vi "CRYGet Curve Library Data Name.vi"(6 "nData":i32[](array[numeric]), 7 "Step No.":i32, 8 "sData":string, 9 "sOption":string, 10 "sAction":string, 11 "Type":enum16{"Curves", "Values", "Results", "WFM"}(ring)) -> (0 "Index":i32[](array[numeric]), 1 "nStep No":i32[](array[numeric]), 2 "sNames":string[](array[string]), 3 "Type Out":string[](array[string]))   [LabVIEW 2013]
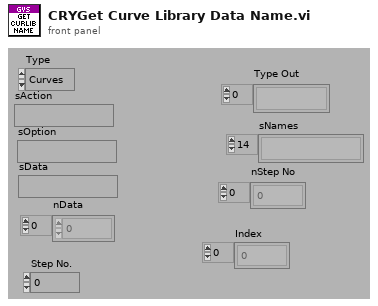
[diagram p1: front panel]
types:
  T1 = typedef "CRYData Cluster.ctl" = cluster{"Name":string, "Curve":cluster{"x":dbl, "y":dbl, "z":dbl}[], "X data":u16, "Y data":u16, "Z data":u16, "X axis":u16, "Y axis":u16, "Z axis":u16, "X unit":string, "Y unit":string, "Z unit":string, "X dB ref":dbl, "Y dB ref":dbl, "Z dB ref":dbl, "single val":bool, "protected":bool, "display X":bool, "display Y":bool, "display Z":bool, "Test Info":string, "Step No.":i32, "Plot Settings":cluster{"Color":u32, "Interpolation":u8, "Point Style":u8, "Line Style":u8, "Point Color":u32, "Line Width":u8, "Bar Plot Style":u8, "Fill To":i16}, "AutoProtect":bool}
  T2 = typedef "CRYWaveform Cluster.ctl" = cluster{"Waveform":cluster{"X0":dbl, "dX":dbl, "Y":sgl[]}, "X data":u16, "Y data":u16, "Y axis":u16, "X unit":string, "Y unit":string, "Y dB ref":dbl, "display Y":bool, "display X":bool, "Overload?":bool, "Test Info":string, "Step No.":i32, "Name":string, "protected":bool, "Sqc history":string[], "Signal Channel ID":i32, "Plot Settings":cluster{"Color":u32, "Interpolation":u8, "Point Style":u8, "Line Style":u8, "Point Color":u32, "Line Width":u8, "Bar Plot Style":u8, "Fill To":i16}, "AutoProtect":bool}
  T3 = typedef "CRYResult Cluster.ctl" = cluster{"Name":string, "Margin":dbl, "unit":string, "Verdict":bool, "Limit":string, "Max/Min":string, "protected":bool, "Step No.":i32, "Test Info":string, "AutoProtect":bool}
  T4 = typedef "CRYStimulus Test Infor Cluster.ctl" = cluster{"Stimulus Type":string, "Signal Type":string, "In/Out":bool, "FAPS":cluster{"freq":dbl, "ampl":dbl, "cycles":dbl, "samples":i32}[], "Sampling Rate":dbl, "Samples":i32, "Analysis Param":string, "Resolution":u16, "Steps":u32, "Analysis Value":dbl[], "Diff Freq":dbl, "FStart":dbl, "FStop":dbl, "Calibration Param":string, "Anti Alias":dbl, "Level Out1":dbl, "Level Out2":dbl, "EQ":bool}
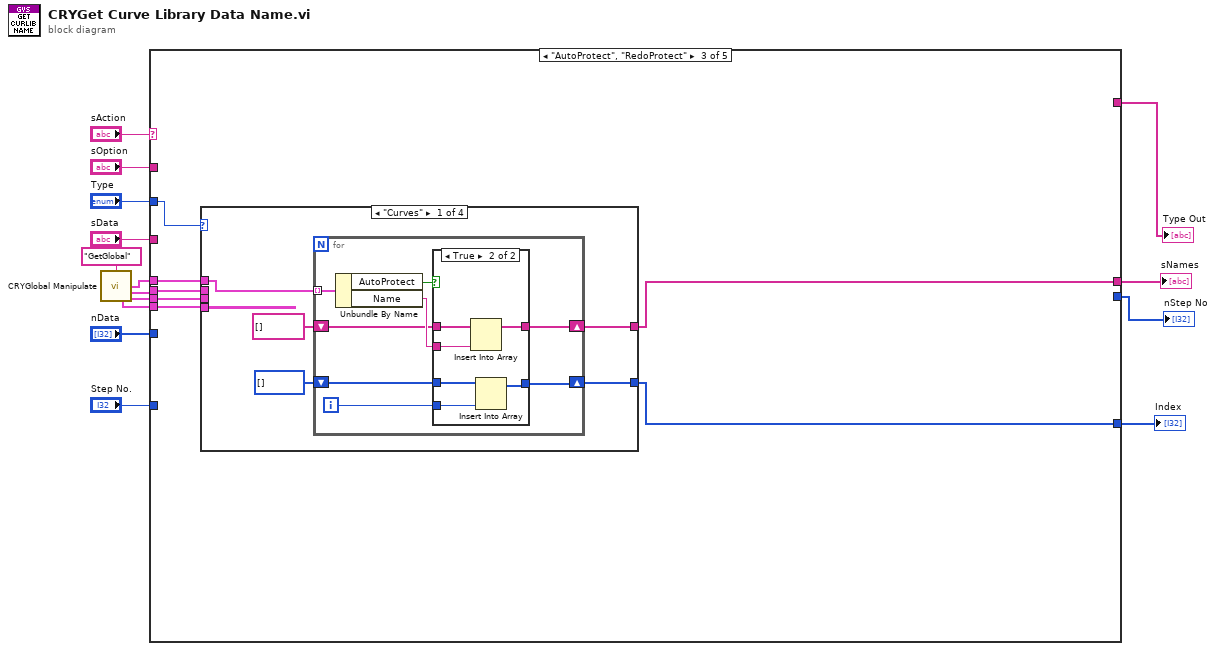
[diagram p0: block diagram]
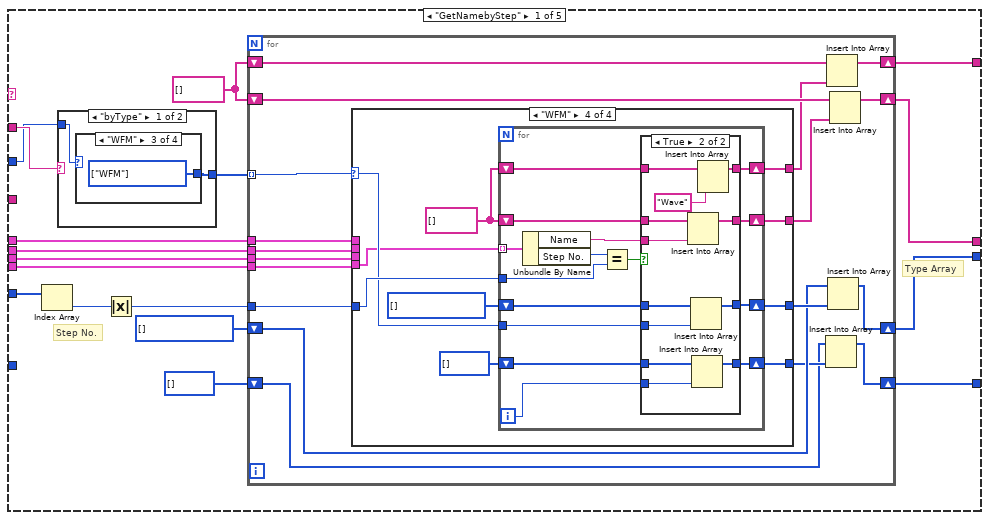
[diagram p2: hidden frame]
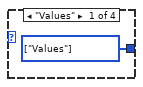
[diagram p3: hidden frame]
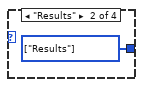
[diagram p4: hidden frame]
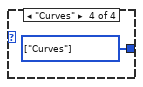
[diagram p5: hidden frame]
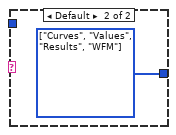
[diagram p6: hidden frame]
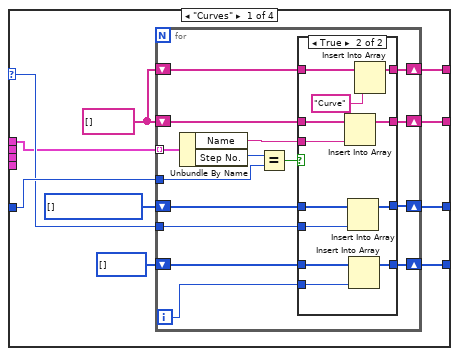
[diagram p7: hidden frame]
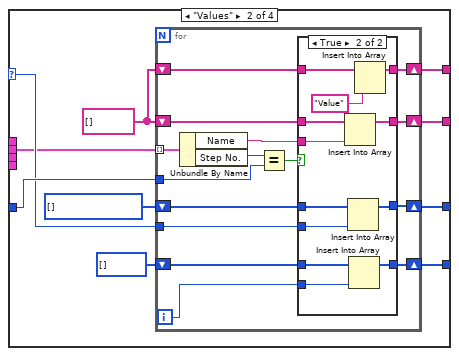
[diagram p9: hidden frame]
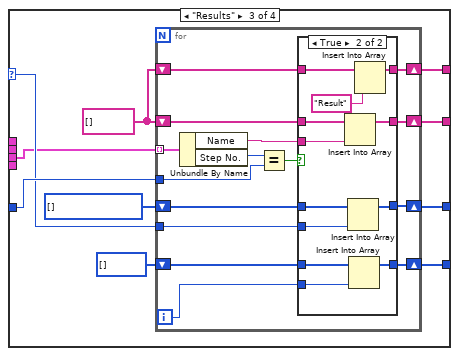
[diagram p11: hidden frame]
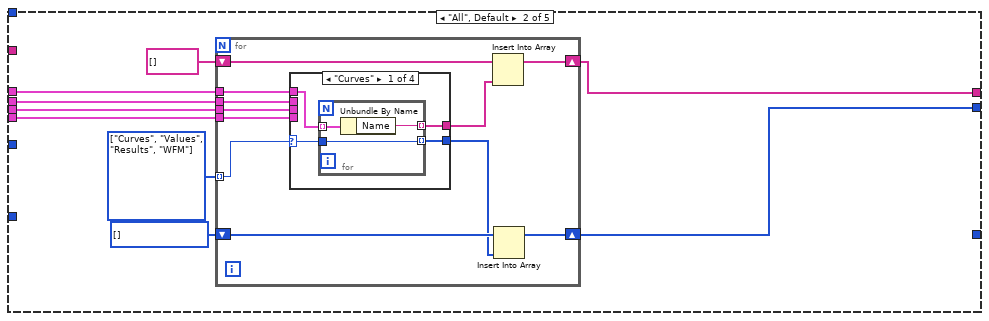
[diagram p14: hidden frame]
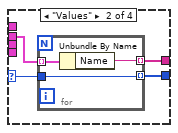
[diagram p15: hidden frame]
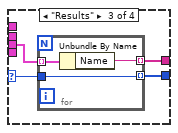
[diagram p16: hidden frame]
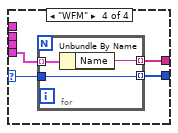
[diagram p17: hidden frame]
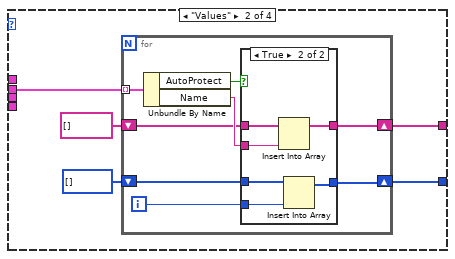
[diagram p19: hidden frame]
diagram:
  n1 = call "CRYGlobal Manipulate.vi"("sAction"="GetGlobal") -> ("Curves Out"=w1:T1[], "Values Out"=w2:T1[], "WFM Out"=w4:T2[], "Results Out"=w5:T3[])  [unwired: 8 in, 3 out]
  n2 = case shown="\"AutoProtect\", \"RedoProtect\"" "sAction" {
    tunnel: "Type" -> [w25 _ w274 _ w532]
    tunnel: "sOption" -> [w26 _ _ _ w536]
    tunnel: "nData" -> [w31 _ _ w367 w531]
    tunnel: "sData" -> [_ _ _ _ w535]
    tunnel: [w29 w228 w275 w368 w534] -> w11
    tunnel: [w27 w226 _ i32[] [] w533] -> w10
    tunnel: [w23 _ w276 _ _] -> w9
    tunnel: "Step No." -> [_ _ _ w366 _]
    tunnel: [w21 _ _ _ _] -> w7
    tunnel: w2 -> [w20 w225 w273 w365 w530]
    tunnel: w5 -> [w19 w224 w272 w364 w529]
    tunnel: w4 -> [w18 w223 w271 w363 w528]
    tunnel: w1 -> [w17 w222 w270 w362 w527]
    frame "GetNamebyStep" {
      w28 = enum16{"Curves", "Values", "Results", "WFM"}[] [] items=["Curves", "Values", "Results", "WFM"]
      w22 = string[] []
      # "Type Array"
      # "Step No."
      n3 = Index Array(array=w31) -> (element=w30:i32)  [unwired: 1 in]
      n4 = case shown="\"byType\"" w26 {
        tunnel: [w33 w39] -> w32
        tunnel: w25 -> [w34 _]
        frame "byType" {
          n5 = case shown="\"WFM\"" w34 {
            tunnel: [w35 w36 w37 w38] -> w33
            frame "Values" {
              w35 = enum16{"Curves", "Values", "Results", "WFM"}[] [enum."Values"] items=["Curves", "Values", "Results", "WFM"]
            }
            frame "Results" {
              w36 = enum16{"Curves", "Values", "Results", "WFM"}[] [enum."Results"] items=["Curves", "Values", "Results", "WFM"]
            }
            frame "WFM" {
              w37 = enum16{"Curves", "Values", "Results", "WFM"}[] [enum."WFM"] items=["Curves", "Values", "Results", "WFM"]
            }
            frame "Curves" {
              w38 = enum16{"Curves", "Values", "Results", "WFM"}[] [enum."Curves"] items=["Curves", "Values", "Results", "WFM"]
            }
          }
        }
        frame Default {
          w39 = enum16{"Curves", "Values", "Results", "WFM"}[] [enum."Curves", enum."Values", enum."Results", enum."WFM"] items=["Curves", "Values", "Results", "WFM"]
        }
      }
      n6 = Absolute Value(x=w30) -> (abs(x)=w16:i32)
      n7 = for {
        tunnel: w32 -> [w47] mode=indexing
        tunnel: w16 -> [w57]
        shift-right: [w55] -> w29
        shift-left: w22 -> [w56]
        shift-right: [w52] -> w27
        shift-left: w28 -> [w53]
        shift-right: [w51] -> w23
        shift-left: i32[] [] -> [w49]
        shift-right: [w44] -> w21
        shift-left: w22 -> [w46]
        tunnel: w20 -> [w43]
        tunnel: w19 -> [w42]
        tunnel: w18 -> [w41]
        tunnel: w17 -> [w40]
        n8 = case shown="\"WFM\"" w47 {
          selector: w47 -> [w64 w105 w146 w187]
          tunnel: w43 -> [_ w101 _ _]
          tunnel: w42 -> [_ _ w140 _]
          tunnel: w41 -> [_ _ _ w181]
          tunnel: w57 -> [w67 w108 w149 w190]
          tunnel: [w66 w107 w148 w189] -> w48
          tunnel: [w63 w104 w145 w186] -> w54
          tunnel: [w61 w102 w143 w184] -> w50
          tunnel: [w59 w99 w141 w182] -> w45
          tunnel: w40 -> [w58 _ _ _]
          frame "Curves" {
            w65 = enum16{"Curves", "Values", "Results", "WFM"}[] [] items=["Curves", "Values", "Results", "WFM"]
            w60 = string[] []
            n9 = for {
              tunnel: w58 -> [w82] mode=indexing
              tunnel: w67 -> [w80]
              shift-right: [w77] -> w66
              shift-left: w60 -> [w76]
              shift-right: [w74] -> w63
              shift-left: w65 -> [w75]
              tunnel: w64 -> [w73]
              shift-right: [w71] -> w61
              shift-left: i32[] [] -> [w70]
              shift-right: [w68] -> w59
              shift-left: w60 -> [w69]
              i -> [w72]
              n10 = Unbundle By Name(w82) -> ("Name"=w78:string, "Step No."=w81:i32)
              n11 = Equal?(x=w81, y=w80) -> (x = y?=w79:bool)
              n12 = case shown="True" w79 {
                tunnel: w78 -> [_ w98]
                tunnel: [w86 w97] -> w77
                tunnel: w76 -> [w86 w96]
                tunnel: [w85 w94] -> w74
                tunnel: w75 -> [w85 w95]
                tunnel: w73 -> [_ w93]
                tunnel: w72 -> [_ w92]
                tunnel: [w84 w91] -> w71
                tunnel: w70 -> [w84 w90]
                tunnel: w69 -> [w83 w89]
                tunnel: [w83 w87] -> w68
                frame False {
                }
                frame True {
                  n13 = Insert Into Array(array=w96, new element=w98) -> (w97:string[])  [unwired: 1 in]
                  n14 = Insert Into Array(array=w95, new element=w93) -> (w94:enum16{"Curves", "Values", "Results", "WFM"}[])  [unwired: 1 in]
                  n15 = Insert Into Array(array=w90, new element=w92) -> (w91:i32[])  [unwired: 1 in]
                  n16 = Insert Into Array(array=w89, new element="Curve") -> (w87:string[])  [unwired: 1 in]
                }
              }
            }
          }
          frame "Values" {
            w106 = enum16{"Curves", "Values", "Results", "WFM"}[] [] items=["Curves", "Values", "Results", "WFM"]
            w100 = string[] []
            n17 = for {
              tunnel: w101 -> [w123] mode=indexing
              tunnel: w108 -> [w121]
              shift-right: [w118] -> w107
              shift-left: w100 -> [w117]
              shift-right: [w115] -> w104
              shift-left: w106 -> [w116]
              tunnel: w105 -> [w114]
              shift-right: [w112] -> w102
              shift-left: i32[] [] -> [w111]
              shift-right: [w109] -> w99
              shift-left: w100 -> [w110]
              i -> [w113]
              n18 = Unbundle By Name(w123) -> ("Name"=w119:string, "Step No."=w122:i32)
              n19 = Equal?(x=w122, y=w121) -> (x = y?=w120:bool)
              n20 = case shown="True" w120 {
                tunnel: w119 -> [_ w139]
                tunnel: [w127 w138] -> w118
                tunnel: w117 -> [w127 w137]
                tunnel: [w126 w135] -> w115
                tunnel: w116 -> [w126 w136]
                tunnel: w114 -> [_ w134]
                tunnel: w113 -> [_ w133]
                tunnel: [w125 w132] -> w112
                tunnel: w111 -> [w125 w131]
                tunnel: w110 -> [w124 w130]
                tunnel: [w124 w128] -> w109
                frame False {
                }
                frame True {
                  n21 = Insert Into Array(array=w137, new element=w139) -> (w138:string[])  [unwired: 1 in]
                  n22 = Insert Into Array(array=w136, new element=w134) -> (w135:enum16{"Curves", "Values", "Results", "WFM"}[])  [unwired: 1 in]
                  n23 = Insert Into Array(array=w131, new element=w133) -> (w132:i32[])  [unwired: 1 in]
                  n24 = Insert Into Array(array=w130, new element="Value") -> (w128:string[])  [unwired: 1 in]
                }
              }
            }
          }
          frame "Results" {
            w147 = enum16{"Curves", "Values", "Results", "WFM"}[] [] items=["Curves", "Values", "Results", "WFM"]
            w142 = string[] []
            n25 = for {
              tunnel: w140 -> [w164] mode=indexing
              tunnel: w149 -> [w162]
              shift-right: [w159] -> w148
              shift-left: w142 -> [w158]
              shift-right: [w156] -> w145
              shift-left: w147 -> [w157]
              tunnel: w146 -> [w155]
              shift-right: [w153] -> w143
              shift-left: i32[] [] -> [w152]
              shift-right: [w150] -> w141
              shift-left: w142 -> [w151]
              i -> [w154]
              n26 = Unbundle By Name(w164) -> ("Name"=w160:string, "Step No."=w163:i32)
              n27 = Equal?(x=w163, y=w162) -> (x = y?=w161:bool)
              n28 = case shown="True" w161 {
                tunnel: w160 -> [_ w180]
                tunnel: [w168 w179] -> w159
                tunnel: w158 -> [w168 w178]
                tunnel: [w167 w176] -> w156
                tunnel: w157 -> [w167 w177]
                tunnel: w155 -> [_ w175]
                tunnel: w154 -> [_ w174]
                tunnel: [w166 w173] -> w153
                tunnel: w152 -> [w166 w172]
                tunnel: w151 -> [w165 w171]
                tunnel: [w165 w169] -> w150
                frame False {
                }
                frame True {
                  n29 = Insert Into Array(array=w178, new element=w180) -> (w179:string[])  [unwired: 1 in]
                  n30 = Insert Into Array(array=w177, new element=w175) -> (w176:enum16{"Curves", "Values", "Results", "WFM"}[])  [unwired: 1 in]
                  n31 = Insert Into Array(array=w172, new element=w174) -> (w173:i32[])  [unwired: 1 in]
                  n32 = Insert Into Array(array=w171, new element="Result") -> (w169:string[])  [unwired: 1 in]
                }
              }
            }
          }
          frame "WFM" {
            w188 = enum16{"Curves", "Values", "Results", "WFM"}[] [] items=["Curves", "Values", "Results", "WFM"]
            w183 = string[] []
            n33 = for {
              tunnel: w181 -> [w205] mode=indexing
              tunnel: w190 -> [w203]
              shift-right: [w200] -> w189
              shift-left: w183 -> [w199]
              shift-right: [w197] -> w186
              shift-left: w188 -> [w198]
              tunnel: w187 -> [w196]
              shift-right: [w194] -> w184
              shift-left: i32[] [] -> [w193]
              shift-right: [w191] -> w182
              shift-left: w183 -> [w192]
              i -> [w195]
              n34 = Unbundle By Name(w205) -> ("Name"=w201:string, "Step No."=w204:i32)
              n35 = Equal?(x=w204, y=w203) -> (x = y?=w202:bool)
              n36 = case shown="True" w202 {
                tunnel: w201 -> [_ w221]
                tunnel: [w209 w220] -> w200
                tunnel: w199 -> [w209 w219]
                tunnel: [w208 w217] -> w197
                tunnel: w198 -> [w208 w218]
                tunnel: w196 -> [_ w216]
                tunnel: w195 -> [_ w215]
                tunnel: [w207 w214] -> w194
                tunnel: w193 -> [w207 w213]
                tunnel: w192 -> [w206 w212]
                tunnel: [w206 w210] -> w191
                frame False {
                }
                frame True {
                  n37 = Insert Into Array(array=w219, new element=w221) -> (w220:string[])  [unwired: 1 in]
                  n38 = Insert Into Array(array=w218, new element=w216) -> (w217:enum16{"Curves", "Values", "Results", "WFM"}[])  [unwired: 1 in]
                  n39 = Insert Into Array(array=w213, new element=w215) -> (w214:i32[])  [unwired: 1 in]
                  n40 = Insert Into Array(array=w212, new element="Wave") -> (w210:string[])  [unwired: 1 in]
                }
              }
            }
          }
        }
        n41 = Insert Into Array(array=w49, new element=w50) -> (w51:i32[])  [unwired: 1 in]
        n42 = Insert Into Array(array=w46, new element=w45) -> (w44:string[])  [unwired: 1 in]
        n43 = Insert Into Array(array=w53, new element=w54) -> (w52:enum16{"Curves", "Values", "Results", "WFM"}[])  [unwired: 1 in]
        n44 = Insert Into Array(array=w56, new element=w48) -> (w55:string[])  [unwired: 1 in]
      }
    }
    frame "All", Default {
      w227 = enum16{"Curves", "Values", "Results", "WFM"}[] [] items=["Curves", "Values", "Results", "WFM"]
      w230 = enum16{"Curves", "Values", "Results", "WFM"}[] [enum."Curves", enum."Values", enum."Results", enum."WFM"] items=["Curves", "Values", "Results", "WFM"]
      n45 = for {
        tunnel: w230 -> [w236] mode=indexing
        shift-right: [w240] -> w228
        shift-left: string[] [] -> [w241]
        shift-right: [w237] -> w226
        shift-left: w227 -> [w238]
        tunnel: w225 -> [w234]
        tunnel: w224 -> [w233]
        tunnel: w223 -> [w232]
        tunnel: w222 -> [w231]
        n46 = case shown="\"Curves\"" w236 {
          selector: w236 -> [w244 w250 w258 w265]
          tunnel: [w245 w252 w259 w266] -> w239
          tunnel: w234 -> [_ w251 _ _]
          tunnel: w233 -> [_ _ w256 _]
          tunnel: w232 -> [_ _ _ w263]
          tunnel: [w243 w249 w257 w264] -> w235
          tunnel: w231 -> [w242 _ _ _]
          frame "Curves" {
            n47 = for {
              tunnel: w242 -> [w248] mode=indexing
              tunnel: [w247] -> w245 mode=indexing
              tunnel: [w246] -> w243 mode=indexing
              tunnel: w244 -> [w246]
              n48 = Unbundle By Name(w248) -> ("Name"=w247:string)
            }
          }
          frame "Values" {
            n49 = for {
              tunnel: w251 -> [w255] mode=indexing
              tunnel: [w254] -> w252 mode=indexing
              tunnel: [w253] -> w249 mode=indexing
              tunnel: w250 -> [w253]
              n50 = Unbundle By Name(w255) -> ("Name"=w254:string)
            }
          }
          frame "Results" {
            n51 = for {
              tunnel: w256 -> [w262] mode=indexing
              tunnel: [w261] -> w259 mode=indexing
              tunnel: [w260] -> w257 mode=indexing
              tunnel: w258 -> [w260]
              n52 = Unbundle By Name(w262) -> ("Name"=w261:string)
            }
          }
          frame "WFM" {
            n53 = for {
              tunnel: w263 -> [w269] mode=indexing
              tunnel: [w268] -> w266 mode=indexing
              tunnel: [w267] -> w264 mode=indexing
              tunnel: w265 -> [w267]
              n54 = Unbundle By Name(w269) -> ("Name"=w268:string)
            }
          }
        }
        n55 = Insert Into Array(array=w241, new element=w239) -> (w240:string[])  [unwired: 1 in]
        n56 = Insert Into Array(array=w238, new element=w235) -> (w237:enum16{"Curves", "Values", "Results", "WFM"}[])  [unwired: 1 in]
      }
    }
    frame "AutoProtect", "RedoProtect" {
      n57 = case shown="\"Curves\"" w274 {
        tunnel: [w280 w301 w322 w343] -> w276
        tunnel: [w278 w299 w320 w341] -> w275
        tunnel: w273 -> [_ w298 _ _]
        tunnel: w272 -> [_ _ w319 _]
        tunnel: w271 -> [_ _ _ w340]
        tunnel: w270 -> [w277 _ _ _]
        frame "Curves" {
          n58 = for {
            tunnel: w277 -> [w288] mode=indexing
            shift-right: [w285] -> w280
            shift-left: i32[] [] ("Index") -> [w289]
            shift-right: [w283] -> w278
            shift-left: string[] [] -> [w282]
            i -> [w287]
            n59 = Unbundle By Name(w288) -> ("AutoProtect"=w286:bool, "Name"=w284:string)
            n60 = case shown="True" w286 {
              tunnel: w289 -> [w291 w297]
              tunnel: w287 -> [_ w296]
              tunnel: [w291 w295] -> w285
              tunnel: w284 -> [_ w294]
              tunnel: [w290 w293] -> w283
              tunnel: w282 -> [w290 w292]
              frame False {
              }
              frame True {
                n61 = Insert Into Array(array=w292, new element=w294) -> (w293:string[])  [unwired: 1 in]
                n62 = Insert Into Array(array=w297, new element=w296) -> (w295:i32[])  [unwired: 1 in]
              }
            }
          }
        }
        frame "Values" {
          n63 = for {
            tunnel: w298 -> [w309] mode=indexing
            shift-right: [w306] -> w301
            shift-left: i32[] [] ("Index") -> [w310]
            shift-right: [w304] -> w299
            shift-left: string[] [] -> [w303]
            i -> [w308]
            n64 = Unbundle By Name(w309) -> ("AutoProtect"=w307:bool, "Name"=w305:string)
            n65 = case shown="True" w307 {
              tunnel: w310 -> [w312 w318]
              tunnel: w308 -> [_ w317]
              tunnel: [w312 w316] -> w306
              tunnel: w305 -> [_ w315]
              tunnel: [w311 w314] -> w304
              tunnel: w303 -> [w311 w313]
              frame False {
              }
              frame True {
                n66 = Insert Into Array(array=w313, new element=w315) -> (w314:string[])  [unwired: 1 in]
                n67 = Insert Into Array(array=w318, new element=w317) -> (w316:i32[])  [unwired: 1 in]
              }
            }
          }
        }
        frame "Results" {
          n68 = for {
            tunnel: w319 -> [w330] mode=indexing
            shift-right: [w327] -> w322
            shift-left: i32[] [] ("Index") -> [w331]
            shift-right: [w325] -> w320
            shift-left: string[] [] -> [w324]
            i -> [w329]
            n69 = Unbundle By Name(w330) -> ("AutoProtect"=w328:bool, "Name"=w326:string)
            n70 = case shown="True" w328 {
              tunnel: w331 -> [w333 w339]
              tunnel: w329 -> [_ w338]
              tunnel: [w333 w337] -> w327
              tunnel: w326 -> [_ w336]
              tunnel: [w332 w335] -> w325
              tunnel: w324 -> [w332 w334]
              frame False {
              }
              frame True {
                n71 = Insert Into Array(array=w334, new element=w336) -> (w335:string[])  [unwired: 1 in]
                n72 = Insert Into Array(array=w339, new element=w338) -> (w337:i32[])  [unwired: 1 in]
              }
            }
          }
        }
        frame "WFM" {
          n73 = for {
            tunnel: w340 -> [w351] mode=indexing
            shift-right: [w348] -> w343
            shift-left: i32[] [] ("Index") -> [w352]
            shift-right: [w346] -> w341
            shift-left: string[] [] -> [w345]
            i -> [w350]
            n74 = Unbundle By Name(w351) -> ("AutoProtect"=w349:bool, "Name"=w347:string)
            n75 = case shown="True" w349 {
              tunnel: w352 -> [w354 w360]
              tunnel: w350 -> [_ w359]
              tunnel: [w354 w358] -> w348
              tunnel: w347 -> [_ w357]
              tunnel: [w353 w356] -> w346
              tunnel: w345 -> [w353 w355]
              frame False {
              }
              frame True {
                n76 = Insert Into Array(array=w355, new element=w357) -> (w356:string[])  [unwired: 1 in]
                n77 = Insert Into Array(array=w360, new element=w359) -> (w358:i32[])  [unwired: 1 in]
              }
            }
          }
        }
      }
    }
    frame "ExcludeSome" {
      w371 = enum16{"Curves", "Values", "Results", "WFM"}[] [enum."Curves", enum."Values", enum."Results", enum."WFM"] items=["Curves", "Values", "Results", "WFM"]
      # "use in CRYMake Name"
      n78 = Absolute Value(x=w366) -> (abs(x)=w361:i32)
      n79 = for {
        tunnel: w371 -> [w379] mode=indexing
        shift-right: [w381] -> w368
        shift-left: string[] [] -> [w382]
        tunnel: w367 -> [w377]
        tunnel: w361 -> [w378]
        tunnel: w365 -> [w375]
        tunnel: w364 -> [w374]
        tunnel: w363 -> [w373]
        tunnel: w362 -> [w372]
        n80 = Index Array(array=w377) -> (element=w376:i32)  [unwired: 1 in]
        n81 = case shown="\"Curves\"" w379 {
          tunnel: [w388 w424 w460 w496] -> w380
          tunnel: w375 -> [_ w419 _ _]
          tunnel: w374 -> [_ _ w455 _]
          tunnel: w373 -> [_ _ _ w493]
          tunnel: w378 -> [w387 w423 w459 w495]
          tunnel: w376 -> [w384 w420 w456 w491]
          tunnel: w372 -> [w383 _ _ _]
          frame "Curves" {
            n82 = for {
              tunnel: w383 -> [w401] mode=indexing
              tunnel: w387 -> [w399]
              shift-right: [w398] -> w388
              shift-left: string[] [] -> [w396]
              shift-right: [w391] -> _
              shift-left: 0 -> [w390]
              tunnel: w384 -> [w392]
              n83 = Unbundle By Name(w401) -> ("Name"=w397:string, "Step No."=w400:i32, "protected"=w394:bool)
              n84 = Greater?(x=w392, y=w390) -> (0:w389:bool)
              n85 = Equal?(x=w400, y=w399) -> (x = y?=w395:bool)
              n86 = Compound Arithmetic op=AND(w395, invert w394) -> (w393:bool)
              n87 = case shown="True" w393 {
                tunnel: [w403 w409] -> w398
                tunnel: w397 -> [w405 w411]
                tunnel: w396 -> [w404 w410]
                tunnel: [w402 w407] -> w391
                tunnel: w390 -> [w402 w406]
                tunnel: w389 -> [_ w408]
                frame False {
                  n88 = Insert Into Array(array=w404, new element=w405) -> (w403:string[])  [unwired: 1 in]
                }
                frame True {
                  n89 = case shown="False" w408 {
                    tunnel: w411 -> [_ w418]
                    tunnel: w410 -> [w413 w417]
                    tunnel: [w413 w416] -> w409
                    tunnel: [w412 w414] -> w407
                    tunnel: w406 -> [w412 w415]
                    frame False {
                    }
                    frame True {
                      n90 = Insert Into Array(array=w417, new element=w418) -> (w416:string[])  [unwired: 1 in]
                      n91 = Increment(x=w415) -> (x+1=w414:i32)
                    }
                  }
                }
              }
            }
          }
          frame "Values" {
            n92 = for {
              tunnel: w419 -> [w437] mode=indexing
              tunnel: w423 -> [w435]
              shift-right: [w434] -> w424
              shift-left: string[] [] -> [w432]
              shift-right: [w427] -> _
              shift-left: 0 -> [w426]
              tunnel: w420 -> [w428]
              n93 = Unbundle By Name(w437) -> ("Name"=w433:string, "Step No."=w436:i32, "protected"=w430:bool)
              n94 = Greater?(x=w428, y=w426) -> (0:w425:bool)
              n95 = Equal?(x=w436, y=w435) -> (x = y?=w431:bool)
              n96 = Compound Arithmetic op=AND(w431, invert w430) -> (w429:bool)
              n97 = case shown="True" w429 {
                tunnel: [w439 w445] -> w434
                tunnel: w433 -> [w441 w447]
                tunnel: w432 -> [w440 w446]
                tunnel: [w438 w443] -> w427
                tunnel: w426 -> [w438 w442]
                tunnel: w425 -> [_ w444]
                frame False {
                  n98 = Insert Into Array(array=w440, new element=w441) -> (w439:string[])  [unwired: 1 in]
                }
                frame True {
                  n99 = case shown="True" w444 {
                    tunnel: w447 -> [_ w454]
                    tunnel: w446 -> [w449 w453]
                    tunnel: [w449 w452] -> w445
                    tunnel: [w448 w450] -> w443
                    tunnel: w442 -> [w448 w451]
                    frame False {
                    }
                    frame True {
                      n100 = Insert Into Array(array=w453, new element=w454) -> (w452:string[])  [unwired: 1 in]
                      n101 = Increment(x=w451) -> (x+1=w450:i32)
                    }
                  }
                }
              }
            }
          }
          frame "Results" {
            n102 = for {
              tunnel: w455 -> [w473] mode=indexing
              tunnel: w459 -> [w471]
              shift-right: [w470] -> w460
              shift-left: string[] [] -> [w468]
              shift-right: [w463] -> _
              shift-left: 0 -> [w462]
              tunnel: w456 -> [w464]
              n103 = Unbundle By Name(w473) -> ("Name"=w469:string, "Step No."=w472:i32, "protected"=w466:bool)
              n104 = Greater?(x=w464, y=w462) -> (0:w461:bool)
              n105 = Equal?(x=w472, y=w471) -> (x = y?=w467:bool)
              n106 = Compound Arithmetic op=AND(w467, invert w466) -> (w465:bool)
              n107 = case shown="True" w465 {
                tunnel: [w475 w481] -> w470
                tunnel: w469 -> [w477 w483]
                tunnel: w468 -> [w476 w482]
                tunnel: [w474 w479] -> w463
                tunnel: w462 -> [w474 w478]
                tunnel: w461 -> [_ w480]
                frame False {
                  n108 = Insert Into Array(array=w476, new element=w477) -> (w475:string[])  [unwired: 1 in]
                }
                frame True {
                  n109 = case shown="True" w480 {
                    tunnel: w483 -> [_ w490]
                    tunnel: w482 -> [w485 w489]
                    tunnel: [w485 w488] -> w481
                    tunnel: [w484 w486] -> w479
                    tunnel: w478 -> [w484 w487]
                    frame False {
                    }
                    frame True {
                      n110 = Insert Into Array(array=w489, new element=w490) -> (w488:string[])  [unwired: 1 in]
                      n111 = Increment(x=w487) -> (x+1=w486:i32)
                    }
                  }
                }
              }
            }
          }
          frame "WFM" {
            n112 = for {
              tunnel: w493 -> [w509] mode=indexing
              tunnel: w495 -> [w507]
              shift-right: [w506] -> w496
              shift-left: string[] [] -> [w504]
              shift-right: [w499] -> _
              shift-left: 0 -> [w498]
              tunnel: w491 -> [w500]
              n113 = Unbundle By Name(w509) -> ("Name"=w505:string, "Step No."=w508:i32, "protected"=w502:bool)
              n114 = Greater?(x=w500, y=w498) -> (0:w497:bool)
              n115 = Equal?(x=w508, y=w507) -> (x = y?=w503:bool)
              n116 = Compound Arithmetic op=AND(w503, invert w502) -> (w501:bool)
              n117 = case shown="True" w501 {
                tunnel: [w511 w517] -> w506
                tunnel: w505 -> [w513 w519]
                tunnel: w504 -> [w512 w518]
                tunnel: [w510 w515] -> w499
                tunnel: w498 -> [w510 w514]
                tunnel: w497 -> [_ w516]
                frame False {
                  n118 = Insert Into Array(array=w512, new element=w513) -> (w511:string[])  [unwired: 1 in]
                }
                frame True {
                  n119 = case shown="True" w516 {
                    tunnel: w519 -> [_ w526]
                    tunnel: w518 -> [w521 w525]
                    tunnel: [w521 w524] -> w517
                    tunnel: [w520 w522] -> w515
                    tunnel: w514 -> [w520 w523]
                    frame False {
                    }
                    frame True {
                      n120 = Insert Into Array(array=w525, new element=w526) -> (w524:string[])  [unwired: 1 in]
                      n121 = Increment(x=w523) -> (x+1=w522:i32)
                    }
                  }
                }
              }
            }
          }
        }
        n122 = Insert Into Array(array=w382, new element=w380) -> (w381:string[])  [unwired: 1 in]
      }
    }
    frame "GetNameByType" {
      n123 = case shown="\"All\", Default" w536 {
        tunnel: w532 -> [w541 w598]
        tunnel: w531 -> [_ w597]
        tunnel: w535 -> [w544 w599]
        tunnel: [w543 w601] -> w534
        tunnel: [w542 w600] -> w533
        tunnel: w530 -> [w540 w596]
        tunnel: w529 -> [w539 w595]
        tunnel: w528 -> [w538 w594]
        tunnel: w527 -> [w537 w593]
        frame "All", Default {
          n124 = case shown="\"WFM\"" w541 {
            tunnel: [w547 w553 w559 w568] -> w543
            tunnel: [w546 w552 w558 w567] -> w542
            tunnel: w544 -> [_ _ _ w564]
            tunnel: w540 -> [_ w551 _ _]
            tunnel: w539 -> [_ _ w557 _]
            tunnel: w538 -> [_ _ _ w563]
            tunnel: w537 -> [w545 _ _ _]
            frame "Curves" {
              n125 = for {
                tunnel: w545 -> [w550] mode=indexing
                tunnel: [w549] -> w547 mode=indexing
                tunnel: [w548] -> w546 mode=indexing
                n126 = Unbundle By Name(w550) -> ("Name"=w549:string, "Step No."=w548:i32)
              }
            }
            frame "Values" {
              n127 = for {
                tunnel: w551 -> [w556] mode=indexing
                tunnel: [w555] -> w553 mode=indexing
                tunnel: [w554] -> w552 mode=indexing
                n128 = Unbundle By Name(w556) -> ("Name"=w555:string, "Step No."=w554:i32)
              }
            }
            frame "Results" {
              n129 = for {
                tunnel: w557 -> [w562] mode=indexing
                tunnel: [w561] -> w559 mode=indexing
                tunnel: [w560] -> w558 mode=indexing
                n130 = Unbundle By Name(w562) -> ("Name"=w561:string, "Step No."=w560:i32)
              }
            }
            frame "WFM" {
              n131 = for {
                tunnel: w563 -> [w584] mode=indexing
                shift-right: [w575] -> w567
                shift-left: i32[] [] -> [w576]
                shift-right: [w574] -> w568
                shift-left: string[] [] -> [w579]
                tunnel: w564 -> [w572]
                n132 = Unbundle By Name(w584) -> ("Name"=w578:string, "Step No."=w577:i32, "Test Info"=w580:string)
                n133 = call "CRYUnflatten Test Infor.vi"("Falattend test infor"=w580) -> ("unflattened test infor data"=w581:T4)  [unwired: 9 out]
                n134 = Unbundle By Name(w581) -> ("Stimulus Type"=w582:string)
                n135 = Equal?(x="ExistType", y=w572) -> (x = y?=w571:bool)
                n136 = Equal?(x=w582, y="") -> (x = y?=w570:bool)
                n137 = And(x=w571, y=w570) -> (x .and. y?=w569:bool)
                n138 = case shown="True" w569 {
                  tunnel: w578 -> [w590 _]
                  tunnel: w579 -> [w589 w592]
                  tunnel: [w588 w592] -> w574
                  tunnel: w577 -> [w587 _]
                  tunnel: w576 -> [w586 w591]
                  tunnel: [w585 w591] -> w575
                  frame False {
                    n139 = Build Array (concatenate)(w586, w587) -> (w585:i32[])
                    n140 = Build Array (concatenate)(w589, w590) -> (w588:string[])
                  }
                  frame True {
                  }
                }
              }
            }
          }
        }
        frame "Some" {
          n141 = case shown="\"Curves\", Default" w598 {
            tunnel: [w605 w614 w623 w635] -> w601
            tunnel: [w604 w613 w622 w634] -> w600
            tunnel: w597 -> [w603 w612 w621 w633]
            tunnel: w599 -> [_ _ _ w630]
            tunnel: w596 -> [_ w611 _ _]
            tunnel: w595 -> [_ _ w620 _]
            tunnel: w594 -> [_ _ _ w629]
            tunnel: w593 -> [w602 _ _ _]
            frame "Curves", Default {
              n142 = for {
                tunnel: w603 -> [w609] mode=indexing
                tunnel: w602 -> [w610]
                tunnel: [w607] -> w605 mode=indexing
                tunnel: [w606] -> w604 mode=indexing
                n143 = Index Array(array=w610, index=w609) -> (element=w608:T1)
                n144 = Unbundle By Name(w608) -> ("Name"=w607:string, "Step No."=w606:i32)
              }
            }
            frame "Values" {
              n145 = for {
                tunnel: w612 -> [w618] mode=indexing
                tunnel: w611 -> [w619]
                tunnel: [w616] -> w614 mode=indexing
                tunnel: [w615] -> w613 mode=indexing
                n146 = Index Array(array=w619, index=w618) -> (element=w617:T1)
                n147 = Unbundle By Name(w617) -> ("Name"=w616:string, "Step No."=w615:i32)
              }
            }
            frame "Results" {
              n148 = for {
                tunnel: w621 -> [w627] mode=indexing
                tunnel: w620 -> [w628]
                tunnel: [w625] -> w623 mode=indexing
                tunnel: [w624] -> w622 mode=indexing
                n149 = Index Array(array=w628, index=w627) -> (element=w626:T3)
                n150 = Unbundle By Name(w626) -> ("Name"=w625:string, "Step No."=w624:i32)
              }
            }
            frame "WFM" {
              n151 = for {
                tunnel: w633 -> [w652] mode=indexing
                tunnel: w629 -> [w653]
                tunnel: w630 -> [w641]
                shift-right: [w643] -> w635
                shift-left: string[] [] -> [w644]
                shift-right: [w638] -> w634
                shift-left: u16[] [] -> [w639]
                n152 = Index Array(array=w653, index=w652) -> (element=w651:T2)
                n153 = Unbundle By Name(w651) -> ("Name"=w645:string, "Step No."=w640:i32, "Test Info"=w637:string)
                n154 = call "CRYUnflatten Test Infor.vi"("Falattend test infor"=w637) -> ("unflattened test infor data"=w650:T4)  [unwired: 9 out]
                n155 = Unbundle By Name(w650) -> ("Stimulus Type"=w649:string)
                n156 = Equal?(x="ExistType", y=w641) -> (x = y?=w647:bool)
                n157 = Equal?(x=w649, y="") -> (x = y?=w646:bool)
                n158 = And(x=w647, y=w646) -> (x .and. y?=w642:bool)
                n159 = case shown="False" w642 {
                  tunnel: w645 -> [w659 _]
                  tunnel: w644 -> [w658 w661]
                  tunnel: [w657 w661] -> w643
                  tunnel: w640 -> [w656 _]
                  tunnel: w639 -> [w655 w660]
                  tunnel: [w654 w660] -> w638
                  frame False {
                    n160 = Build Array (concatenate)(w655, w656) -> (w654:i32[])
                    n161 = Build Array (concatenate)(w658, w659) -> (w657:string[])
                  }
                  frame True {
                  }
                }
              }
            }
          }
        }
      }
    }
  }
  "sNames" <- w11
  "nStep No" <- w10
  "Index" <- w9
  "Type Out" <- w7
